vi "connect_with_last_node_term.vi"(7 "Last StrCnst Refnum":refnum<vi>, 8 "error in (no error)":errorcluster, 9 "Terminal Index":T1 items=["AppendTrueFalseString/VisaWrite"=4, "PickLine"=3, "FormatIntoString/Concatenate"=1], 10 "Terminals[]":refnum<vi>[](array[refnum]), 11 "Last Function Ref In":refnum<vi>) -> (0 "error out":errorcluster)   [LabVIEW 2018]
uses:
  TypeDefines/connect_with_last_node_types.ctl
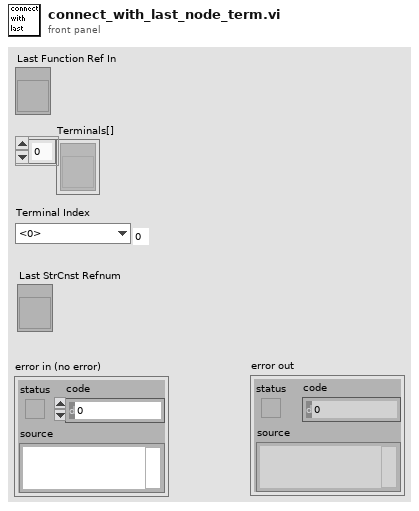
[diagram p1: front panel]
types:
  T1 = typedef "connect_with_last_node_types.ctl" = u16
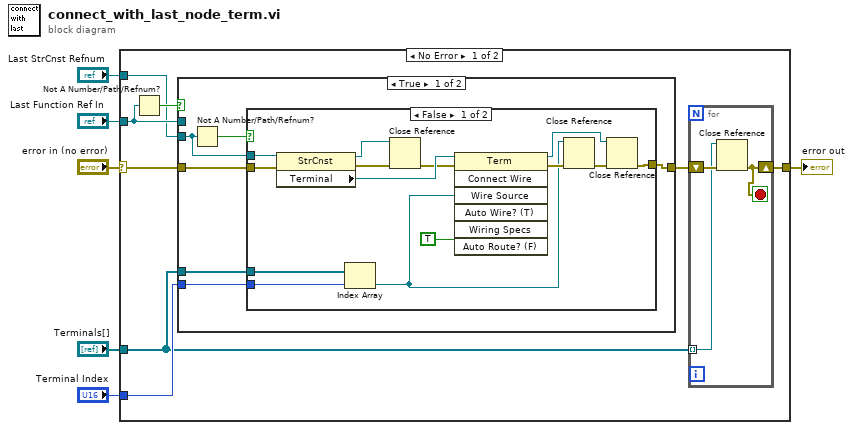
[diagram p0: block diagram]
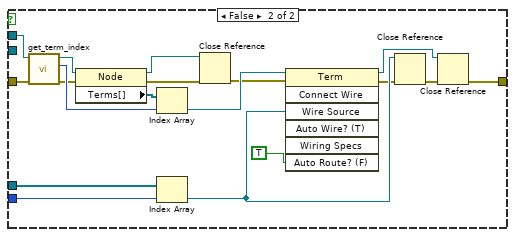
[diagram p3: hidden frame]
diagram:
  n1 = case shown="No Error" "error in (no error)" {
    selector: "error in (no error)" -> [w13 w57]
    tunnel: "Last Function Ref In" -> [w12 _]
    tunnel: [w9 w57] -> w4
    tunnel: "Terminals[]" -> [w8 _]
    tunnel: "Terminal Index" -> [w11 _]
    tunnel: "Last StrCnst Refnum" -> [w7 _]
    frame No Error {
      n2 = Not A Number/Path/Refnum?(number/path/refnum=w12) -> (NaN/Path/Refnum?=w14:bool)
      n3 = case shown="True" w14 {
        tunnel: w12 -> [_ w56]
        tunnel: w8 -> [w22 w52]
        tunnel: [w18 w47] -> w10
        tunnel: w13 -> [w19 w50]
        tunnel: w11 -> [w21 w49]
        tunnel: w7 -> [w20 _]
        frame True {
          n4 = Not A Number/Path/Refnum?(number/path/refnum=w20) -> (NaN/Path/Refnum?=w23:bool)
          n5 = case shown="False" w23 {
            tunnel: w22 -> [w34 _]
            tunnel: w21 -> [w33 _]
            tunnel: w20 -> [w31 _]
            tunnel: w19 -> [w32 w38]
            tunnel: [w27 w38] -> w18
            frame False {
              n6 = property class="StrCnst"(reference=w31, error in=w32) -> (reference out=w26:refnum<vi>, error out=w25:errorcluster, "Terminal"=w30:refnum<vi>)
              n7 = Index Array(array=w34, index=w33) -> (element=w29:refnum<vi>)
              n8 = Close Reference(reference=w26, error in (no error)=w25) -> (error out=w24:errorcluster)
              n9 = invoke class="Term" method="Connect Wire"(reference=w30, error in=w24, "Wire Source"=w29, "Auto Route? (F)"=TRUE) -> (reference out=w36:refnum<vi>, error out=w35:errorcluster)  [unwired: 3 in, 5 out]
              n10 = Close Reference(reference=w29, error in (no error)=w35) -> (error out=w37:errorcluster)
              n11 = Close Reference(reference=w36, error in (no error)=w37) -> (error out=w27:errorcluster)
            }
            frame True {
            }
          }
        }
        frame False {
          n12 = call "get_term_index.vi"("error in (no error)"=w50, "Last Function Ref In"=w56) -> ("error out"=w51:errorcluster, "Term Index"=w53:i32, "Last Function Ref Out"=w54:refnum<vi>)  [unwired: 7 out]
          n13 = property class="Node"(reference=w54, error in=w51) -> (reference out=w41:refnum<vi>, error out=w40:errorcluster, "Terms[]"=w55:refnum<vi>[])
          n14 = Index Array(array=w55, index=w53) -> (element=w48:refnum<vi>)
          n15 = Index Array(array=w52, index=w49) -> (element=w44:refnum<vi>)
          n16 = Close Reference(reference=w41, error in (no error)=w40) -> (error out=w39:errorcluster)
          n17 = invoke class="Term" method="Connect Wire"(reference=w48, error in=w39, "Wire Source"=w44, "Auto Route? (F)"=TRUE) -> (reference out=w45:refnum<vi>, error out=w43:errorcluster)  [unwired: 3 in, 5 out]
          n18 = Close Reference(reference=w44, error in (no error)=w43) -> (error out=w46:errorcluster)
          n19 = Close Reference(reference=w45, error in (no error)=w46) -> (error out=w47:errorcluster)
        }
      }
      n20 = for {
        shift-right: [w15] -> w9
        shift-left: w10 -> [w17]
        tunnel: w8 -> [w16] mode=indexing
        stop <- w15 stop-if-true
        n21 = Close Reference(reference=w16, error in (no error)=w17) -> (error out=w15:errorcluster)
      }
    }
    frame Error {
    }
  }
  "error out" <- w4
